vi "kA to Tesla v0.80.vi"(3 "kA":dbl=36.0 format="%.2f", 4 "Magnet ID":i32(ring)=7 items=["None", "Cell 12", "Cell 3 A", "Cell 3 B", "Cell 3", "Cell 4", "Cell 4-2", "Cell 4-3", "Cell 5", "Cell 6-2", "Cell 6-3", "Cell 7", "Cell 8", "Cell 9", "SCM1", "SCM2"]) -> (0 "Calibration":T1={"Current Scale Factor kA/V"=1.0, "I->B"=[0.0, 1.0, 0.0], "B->I"=[0.0, 1.0, 0.0]} {"B->I" format="%.5e"; "Current Scale Factor kA/V" format="%.2f"; "I->B" format="%.5e"}, 1 "Magnetic Field (T)":dbl format="%.2f")   [LabVIEW 2025]
doc: "Author: Scott Hannahs <sth@magnet.fsu.edu>\n\nThis software is licensed for use under the “MIT License\"\nCopyright (c) 2025 Scott Hannahs, sth@sth@magnet.sthnet.net\n\nPermission is hereby granted, free of charge, to any person obtaining a copy of this software and associated documentation files (the \"Software\"), to deal in the Software without restriction, including without limitation the rights to use, copy, modify, merge, publish, distribute, sublicense, and/or sell copies of the Software, and to permit persons to whom the Software is furnished to do so, subject to the following conditions: The above copyright notice and this permission notice shall be included in all copies or substantial portions of the Software.\n\nTHE SOFTWARE IS PROVIDED \"AS IS\", WITHOUT WARRANTY OF ANY KIND, EXPRESS OR IMPLIED, INCLUDING BUT NOT LIMITED TO THE WARRANTIES OF MERCHANTABILITY, FITNESS FOR A PARTICULAR PURPOSE AND NONINFRINGEMENT. IN NO EVENT SHALL THE AUTHORS OR COPYRIGHT HOLDERS BE LIABLE FOR ANY CLAIM, DAMAGES OR OTHER LIABILITY, WHETHER IN AN ACTION OF CONTRACT, TORT OR OTHERWISE, ARISING FROM, OUT OF OR IN CONNECTION WITH THE SOFTWARE OR THE USE OR OTHER DEALINGS IN THE SOFTWARE."
panel:
  out "Voltage output":dbl=9.0 format="%.4f"
  in  "Field input":dbl=30.7082 format="%.2f"
  out "kA output":dbl=35.99847519140809 format="%.5f"
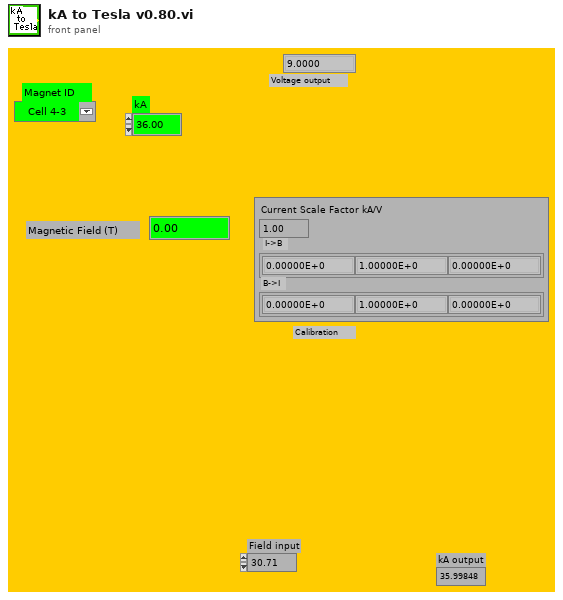
[diagram p1: front panel]
types:
  T1 = cluster{"Current Scale Factor kA/V":dbl, "I->B":dbl[], "B->I":dbl[]}
  T2 = cluster{"I->B[0]":dbl, "I->B[1]":dbl, "I->B[2]":dbl}
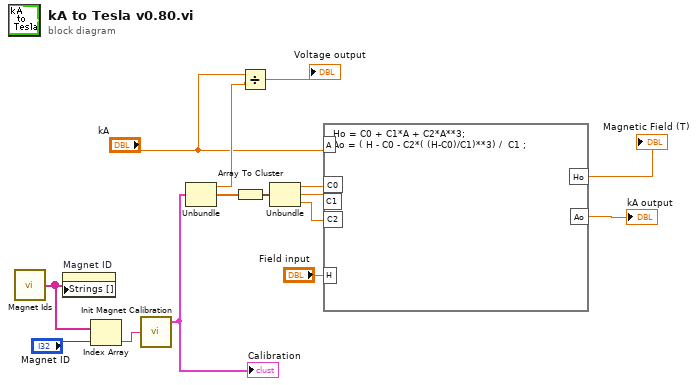
[diagram p0: block diagram]
diagram:
  n1 = call "Magnet Ids.vi"() -> ("Magnet IDs"=w2:string[])
  n2 = property on="Magnet ID" class="Ring (strict)"("Strings []"=w2) -> ()  [unwired: 2 in, 2 out]
  n3 = Index Array(array=w2, index="Magnet ID") -> (element=w14:string)
  n4 = call "Init Magnet Calibration.vi"("Magnet Id"=w14) -> ("Calibration"=w1:T1)  [unwired: 2 out]
  "Calibration" <- w1
  n5 = Unbundle(w1) -> ("Current Scale Factor kA/V"=w5:dbl, "I->B"=w12:dbl[])  [unwired: 1 out]
  n6 = Array To Cluster(array=w12) -> (cluster=w13:T2)
  n7 = Divide(x="kA", y=w5) -> (x/y=→"Voltage output":dbl)
  n8 = Unbundle(w13) -> ("I->B[0]"=w11:dbl, "I->B[1]"=w10:dbl, "I->B[2]"=w9:dbl)
  n9 = formula code="Ho = C0 + C1*A + C2*A**3;\nAo = ( H - C0 - C2*( (H-C0)/C1)**3) /  C1 ;"("C0"=w11, "C1"=w10, "C2"=w9, "A"="kA", "H"="Field input") -> ("Ho"=→"Magnetic Field (T)":dbl, "Ao"=→"kA output":dbl)
